vi "一体站流程自动启动.vi"(11 "参数":T1={"是否启用仪器"=FALSE, "CODMn"={"启动测量模式"={"测量模式"=enum."水样测量"}, "确定按钮"=TRUE}, "CODCr"={"启动测量模式"={"测量模式"=enum."水样测量"}}, "采水模式"=enum."使用采水泵"}) -> ()   [LabVIEW 2016, in "PLC.lvlib"]
uses:
  PLC.lvlib
  API/CodCr/CodCr.lvlib
panel:
  out "枚举":enum16{"初始化", "采配水启动", "等待", "配水", "排水", "结束"}(ring)
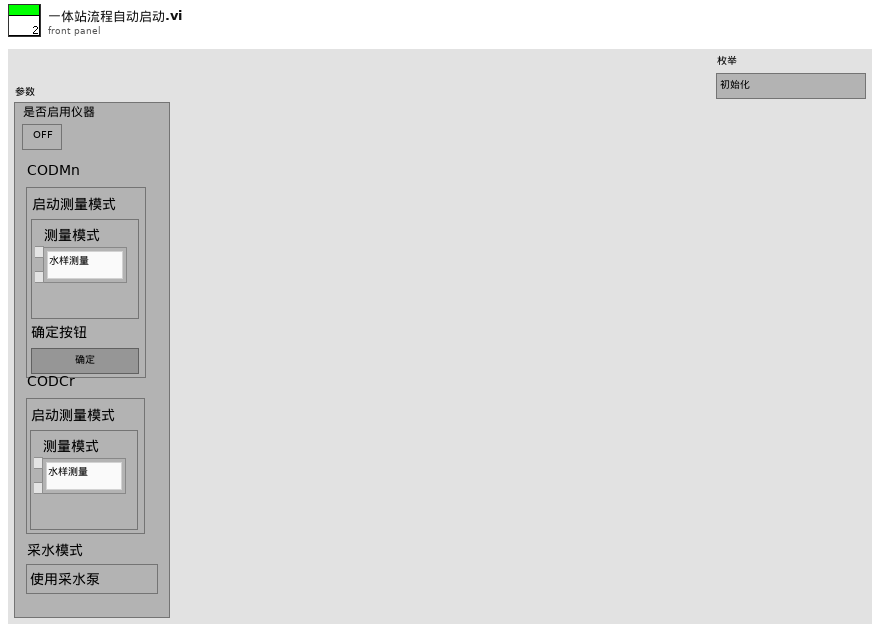
[diagram p1: front panel]
types:
  T1 = cluster{"是否启用仪器":bool, "CODMn":cluster{"启动测量模式":cluster{"测量模式":enum16{"水样测量", "标样核查", "零点核查", "加标回收", "平行样", "校零", "校标"}}, "确定按钮":bool}, "CODCr":cluster{"启动测量模式":cluster{"测量模式":enum16{"水样测量", "标样核查", "零点核查", "加标回收", "平行样", "校零", "校标"}}}, "采水模式":enum16{"使用采水泵", "不使用采水泵"}}
  T2 = cluster{"命令":string, cluster{"starting address":u16, "holding register value":u16}}
  T3 = enum16{"待机", "启动氨氮", "氨氮测量中", "启动总磷", "总磷测量中", "结束"}
  T4 = enum16{"空闲", "水样测试", "标样核查", "零点核查", "跨度核查", "空白测试", "平行样测试", "加标回收", "空白校准", "标样校准", "初始化（清洗）"}
  T5 = cluster{"站号":u16, "量程切换":enum32{"H", "L", "AUTO"}, "控制命令":enum16{"启动测量", "标样核查", "零点核查", "跨度核查", "空白测试", "平行样测试", "加标回收", "空白校准", "标样校准", "初始化（清洗）", "停止测试", "仪器重启", "校时", "模式设置", "测量间隔设置", "盲样测试"}, "模式设置":enum16{"待机", "连续模式", "周期模式", "定点模式", "受控模式", "手动模式"}, "测量间隔":u16}
  T6 = cluster{"时间标识":timestamp, "设备":string, "日志信息":string}
  T7 = cluster{"测试时间":dbl, "运行模式":enum16{"维护模式", "常规模式", "应急模式", "质控模式"}}
  T8 = cluster{"R0":i16, "R1":i16, "R2":i16, "R3":i16, "R4":i16, "R5":i16, "R6":i16, "R7":i16, "R8":i16, "R9":i16, "R10":i16, "R11":i16, "R12":i16, "R13":i16, "R14":i16, "R15":i16, "R16":i16, "R17":i16, "R18":i16, "R19":i16, "R20":i16, "R21":i16}
  T9 = cluster{"测量模式":enum16{"水样测量", "标样核查", "零点核查", "加标回收", "平行样", "校零", "校标"}}
  T10 = enum32{"Bad", "Idle", "Run top level", "Running"}
  T11 = cluster{"系统时间":timestamp, "工作状态":enum16{"空闲", "水样测试", "标样核查", "零点核查", "跨度核查", "空白测试", "平行样测试", "加标回收", "空白校准", "标样校准", "初始化（清洗）"}, "测量模式":enum16{"待机", "连续模式", "周期模式", "定点模式", "受控模式", "手动模式"}, "告警代码":enum16{"无告警", "缺试剂告警", "缺水样告警", "缺蒸馏水告警", "缺标液告警", "仪表漏液告警", "标定异常告警", "超量程告警", "加热异常", "低试剂预警", "超上限告警", "超下限告警", "仪表内部其他异常", "滴定异常告警", "电极异常告警", "量程切换告警", "参数设置告警", "PH电极电位异常", "电导率电极异常", "浊度光度异常", "溶解氧电极异常", "溶解氧光强异常", "温度异常告警", "PH异常告警", "溶解氧异常告警", "电导率异常告警", "浊度异常告警", "叶绿素异常告警", "藻密度异常告警", "蓝绿藻异常告警", "ORP异常告警", "氨氮异常告警", "清洁刷异常告警", "SD卡异常告警", "蓝牙异常告警", "Wifi异常告警", "流程异常告警"}, "故障代码":enum16{"无故障", "电机故障", "温度故障", "通讯故障", "滴定故障"}, "日志代码":u16, "软件版本":u16, "F0":sgl, "F1":sgl, "F2":sgl, "F3":sgl, "T":sgl, "H":sgl, "id":u16, "flowid":u16, "量程":u16}
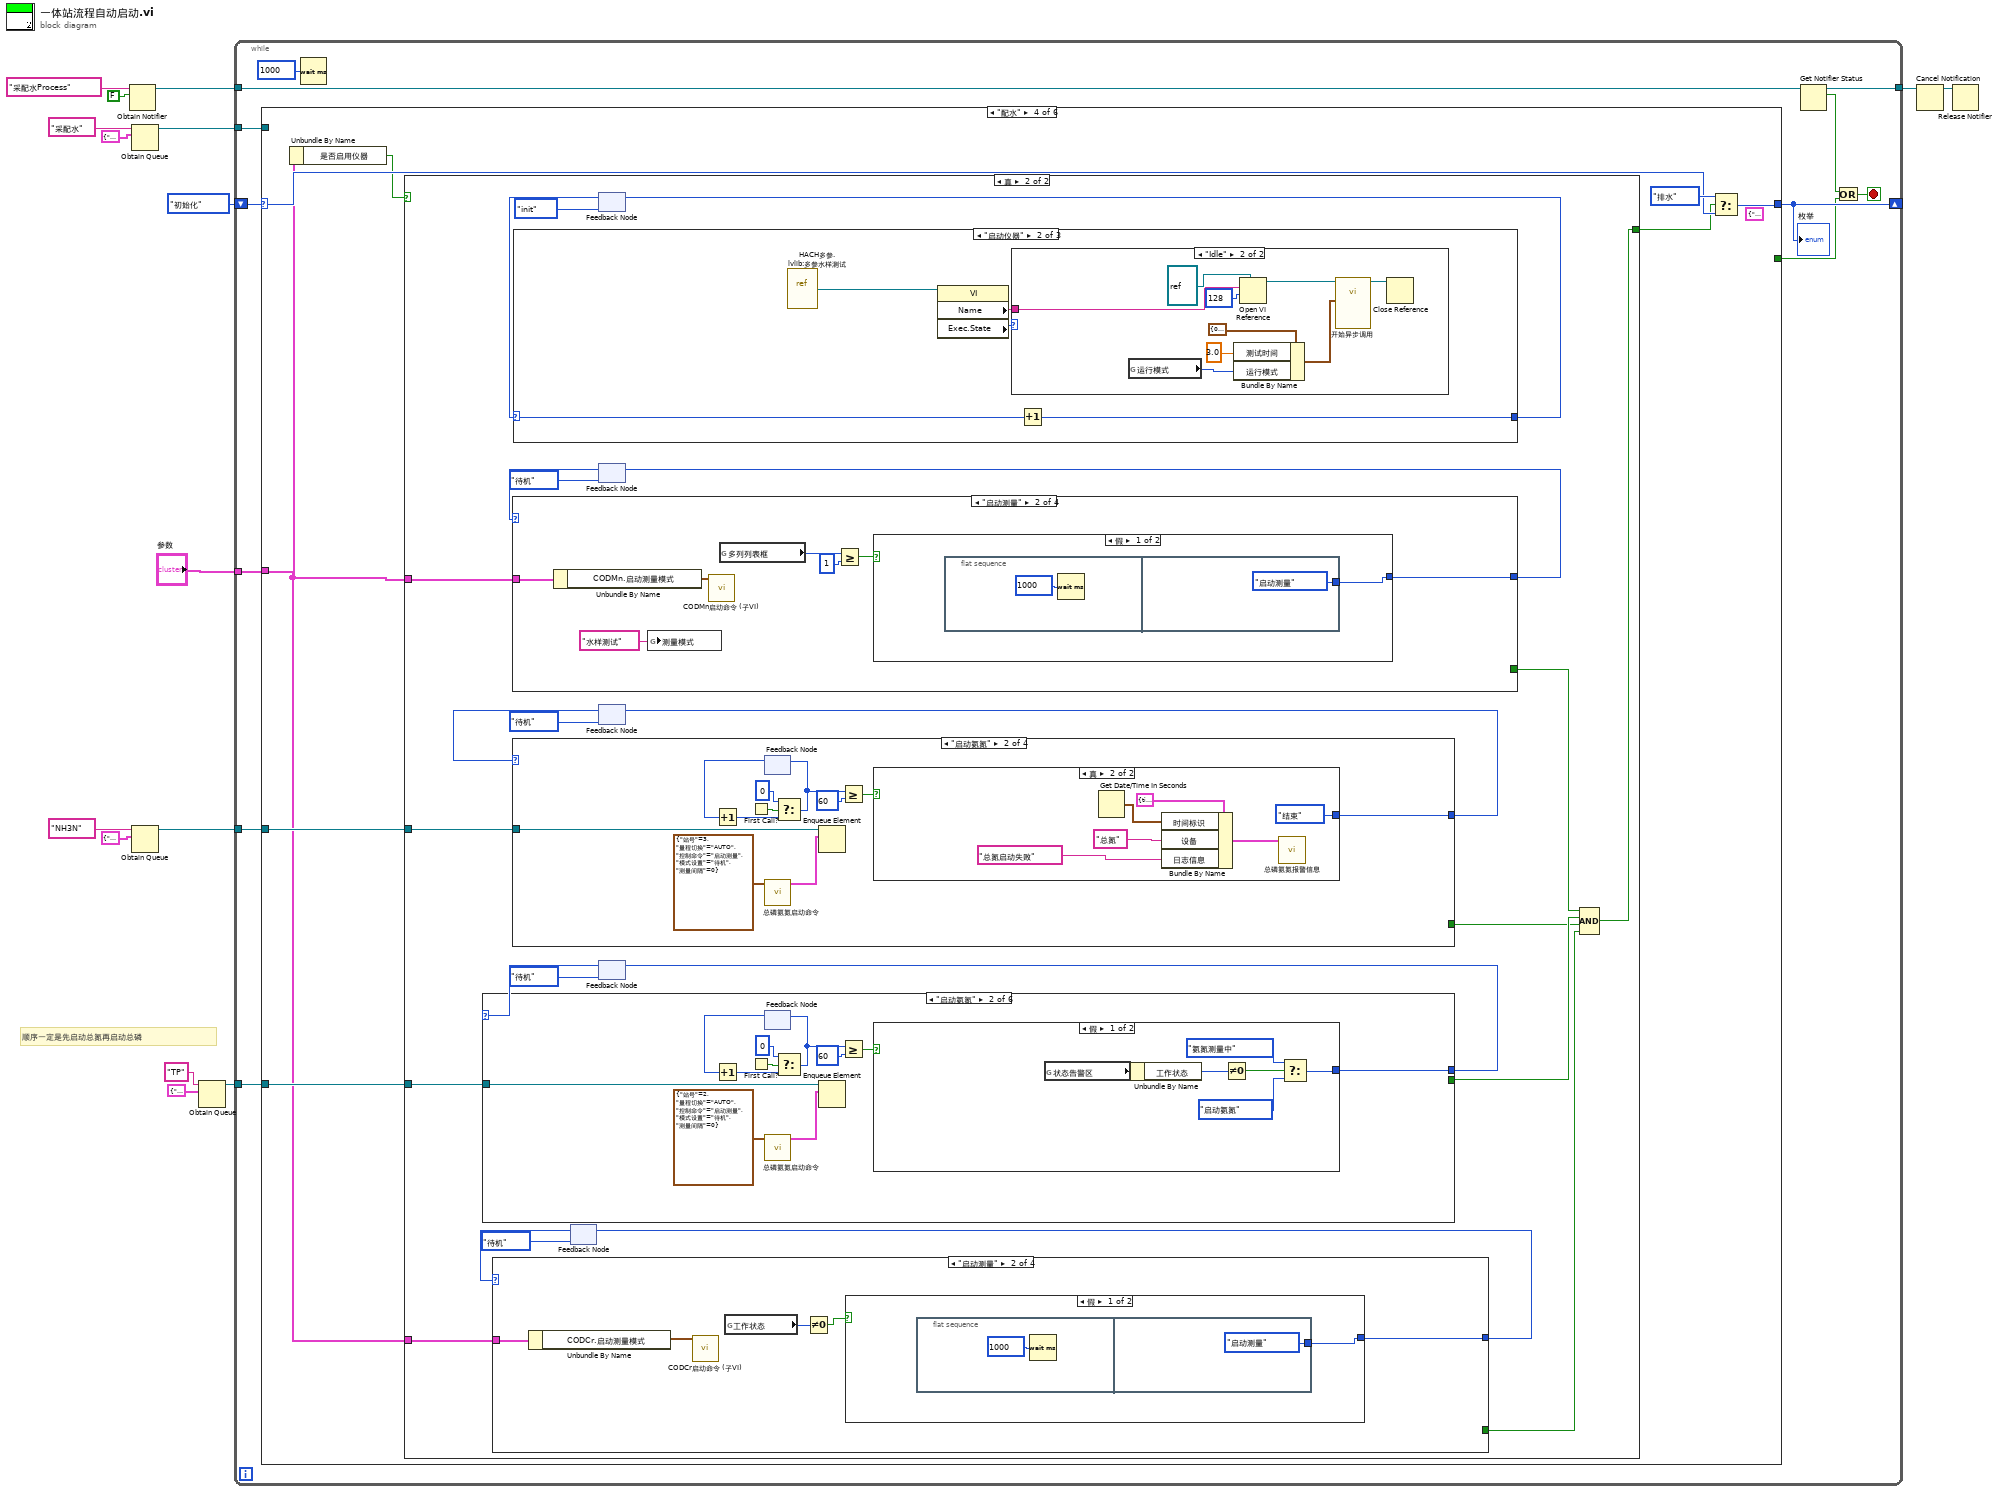
[diagram p0: block diagram]
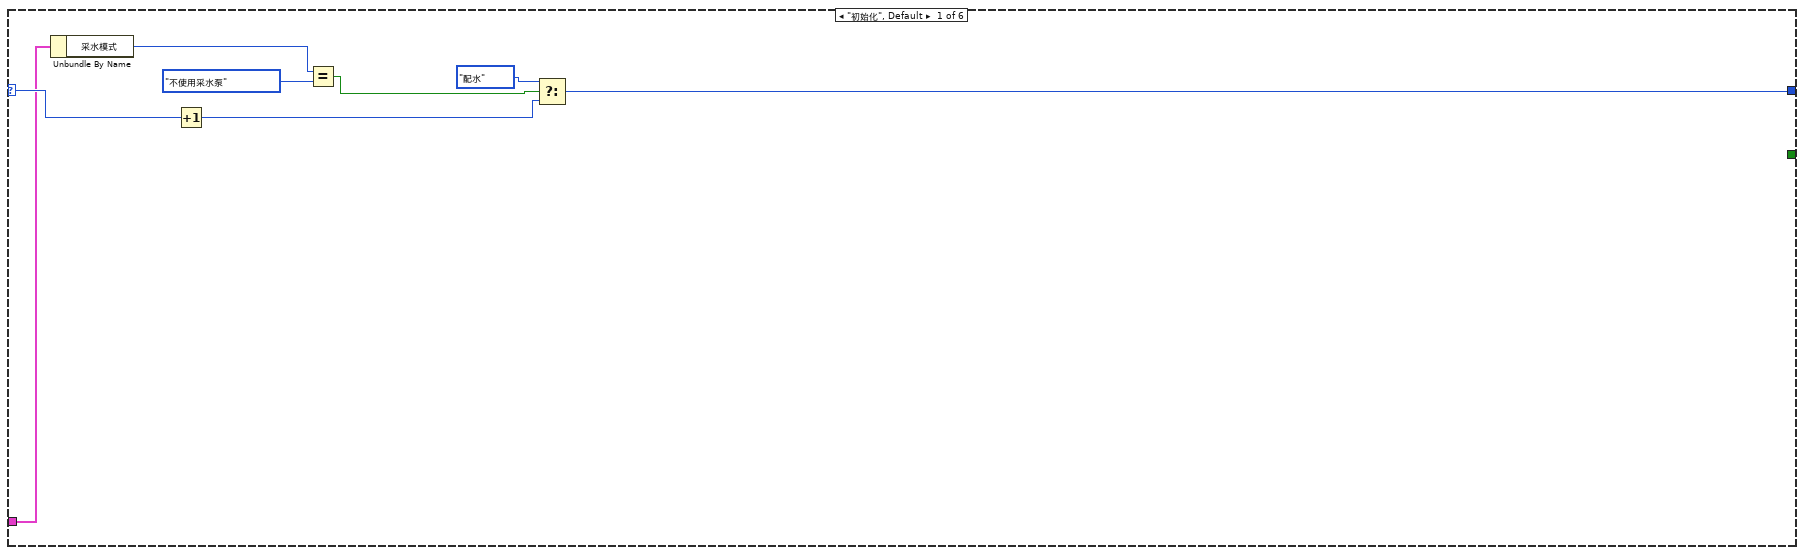
[diagram p2: hidden frame]
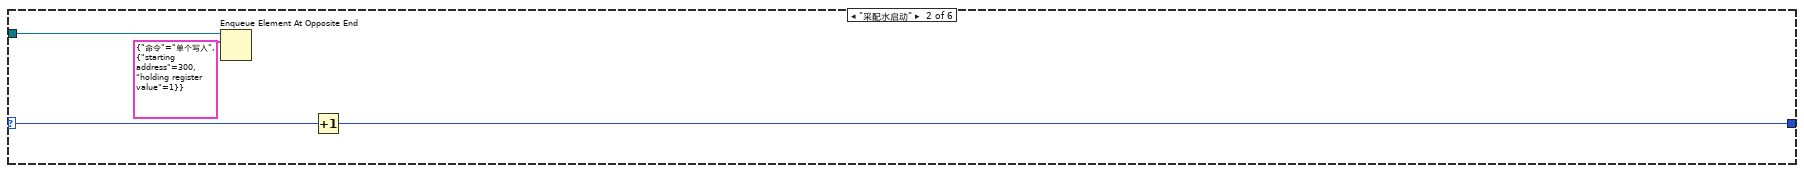
[diagram p3: hidden frame]
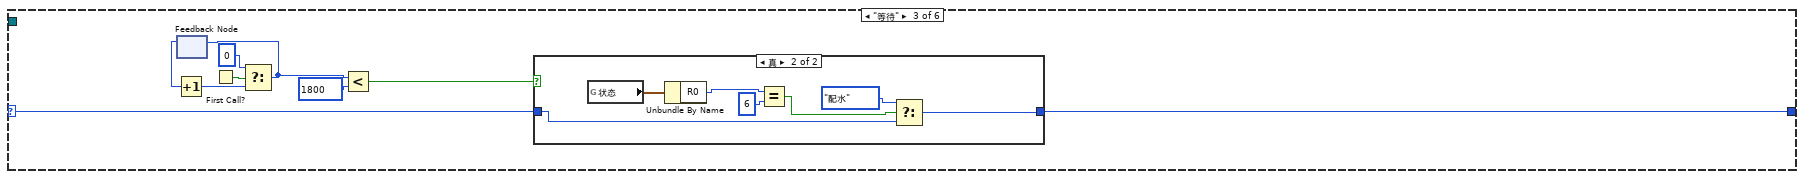
[diagram p4: hidden frame]
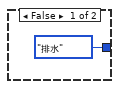
[diagram p5: hidden frame]
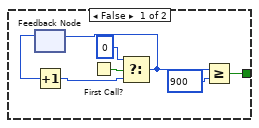
[diagram p6: hidden frame]
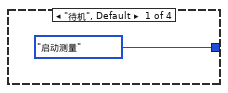
[diagram p7: hidden frame]
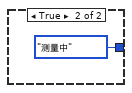
[diagram p8: hidden frame]
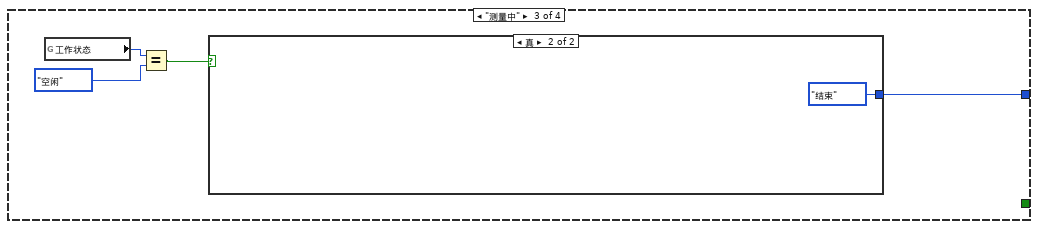
[diagram p9: hidden frame]
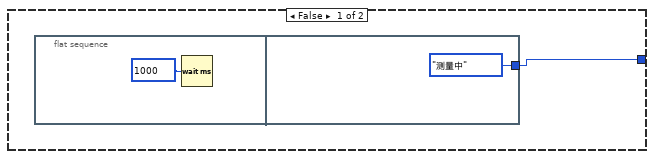
[diagram p10: hidden frame]
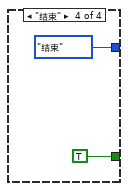
[diagram p11: hidden frame]
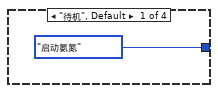
[diagram p12: hidden frame]
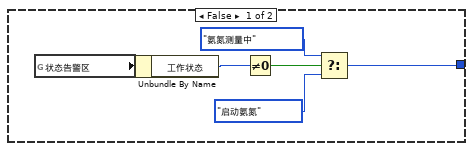
[diagram p13: hidden frame]
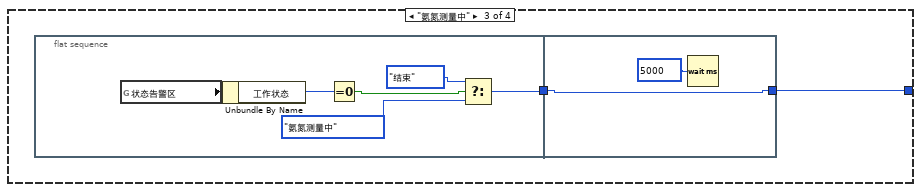
[diagram p14: hidden frame]
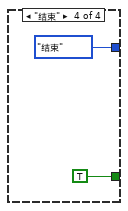
[diagram p15: hidden frame]
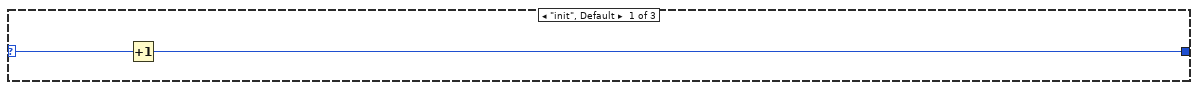
[diagram p16: hidden frame]
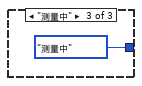
[diagram p18: hidden frame]
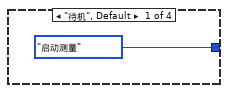
[diagram p19: hidden frame]
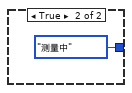
[diagram p20: hidden frame]
diagram:
  # "顺序一定是先启动总氮再启动总磷"
  n1 = Obtain Notifier(name (unnamed)="采配水Process" ("名称（未命名）"), notification data type=FALSE) -> (notifier out=w6:refnum<notifier>)  [unwired: 2 in, 2 out]
  n2 = Obtain Queue(name (unnamed)="采配水" ("名称（未命名）"), element data type=cluster{"命令":string, "数据":variant} {"命令"="", "数据"=variant}) -> (queue out=w14:refnum<queue>)  [unwired: 3 in, 2 out]
  n3 = Obtain Queue(name (unnamed)="NH3N" ("名称（未命名）"), element data type=cluster{"命令":string, "data":variant} {"命令"="", "data"=variant}) -> (queue out=w1:refnum<queue>)  [unwired: 3 in, 2 out]
  n4 = Obtain Queue(name (unnamed)="TP" ("名称（未命名）"), element data type=cluster{"命令":string, "data":variant} {"命令"="", "data"=variant}) -> (queue out=w10:refnum<queue>)  [unwired: 3 in, 2 out]
  n5 = while {
    tunnel: w14 -> [w28]
    shift-right: [w26] -> _
    shift-left: enum16{"初始化", "采配水启动", "等待", "配水", "排水", "结束"}."初始化" ("枚举") -> [w27]
    tunnel: w10 -> [w24]
    tunnel: "参数" -> [w23]
    tunnel: w6 -> [w22]
    tunnel: [w21] -> w5
    tunnel: w1 -> [w17]
    stop <- w20 stop-if-true
    n6 = case shown="\"配水\"" w27 {
      selector: w27 -> [w36 w38 w47 w64 w262 w267]
      tunnel: w28 -> [_ w39 _ _ w263 _]
      tunnel: [w29 w37 w46 w63 w261 w266] -> w26
      tunnel: [_ _ _ _ _ TRUE] -> w19
      tunnel: w24 -> [_ _ _ w62 _ _]
      tunnel: w23 -> [w35 _ _ w58 _ _]
      tunnel: w17 -> [_ _ _ w59 _ _]
      frame "初始化", Default {
        n7 = Unbundle By Name(w35) -> ("采水模式"=w34:enum16{"使用采水泵", "不使用采水泵"})
        n8 = Increment(x=w36) -> (x+1=w30:enum16{"初始化", "采配水启动", "等待", "配水", "排水", "结束"})
        n9 = Equal?(x=w34, y=enum16{"使用采水泵", "不使用采水泵"}."不使用采水泵") -> (x = y?=w32:bool)
        n10 = Select(t=enum16{"初始化", "采配水启动", "等待", "配水", "排水", "结束"}."配水" ("枚举"), s=w32, f=w30) -> (s? t:f=w29:enum16{"初始化", "采配水启动", "等待", "配水", "排水", "结束"})
      }
      frame "采配水启动" {
        n11 = Enqueue Element At Opposite End(queue=w39, element=T2 {"命令"="单个写入", {"starting address"=300, "holding register value"=1}} ("元素")) -> ()  [unwired: 2 in, 3 out]
        n12 = Increment(x=w38) -> (x+1=w37:enum16{"初始化", "采配水启动", "等待", "配水", "排水", "结束"})
      }
      frame "等待" {
        n13 = feedback #1() -> (w43:i32)  [unwired: 1 in]
        n14 = Increment(x=w43) -> (x+1=w42:i32)
        n15 = First Call?() -> (First Call?: T/F=w44:bool)
        n16 = Select(t=0, s=w44, f=w42) -> (s? t:f=w41:i32)
        n17 = feedback-in #1(w41) -> ()
        n18 = Less?(x=w41, y=1800) -> (x < y?=w48:bool)
        n19 = case shown="真" w48 {
          tunnel: w47 -> [_ w52]
          tunnel: [enum16{"初始化", "采配水启动", "等待", "配水", "排水", "结束"}."排水" ("枚举") w51] -> w46
          frame False {
          }
          frame True {
            n20 = global read "采配水全局变量.vi" "状态"() -> (w57:T8)
            n21 = Unbundle By Name(w57) -> ("R0"=w56:i16)
            n22 = Equal?(x=w56, y=i16 6) -> (x = y?=w54:bool)
            n23 = Select(t=enum16{"初始化", "采配水启动", "等待", "配水", "排水", "结束"}."配水" ("枚举"), s=w54, f=w52) -> (s? t:f=w51:enum16{"初始化", "采配水启动", "等待", "配水", "排水", "结束"})
          }
        }
      }
      frame "配水" {
        (unwired) cluster{"命令":string, "data":variant} {"命令"="启动", "data"=variant(cluster{"站号":u16, "控制命令输出":u16[]} {"站号"=1, "控制命令输出"=[256, 0]})} ("元素")
        n24 = Unbundle By Name(w58) -> ("是否启用仪器"=w61:bool)
        n25 = case shown="真" w61 {
          tunnel: w62 -> [_ w93]
          tunnel: [w66 w78] -> w60
          tunnel: w58 -> [_ w89]
          tunnel: w59 -> [_ w82]
          tunnel: w58 -> [_ w74]
          frame False {
            n26 = feedback #2() -> (w70:i32)  [unwired: 1 in]
            n27 = Increment(x=w70) -> (x+1=w69:i32)
            n28 = First Call?() -> (First Call?: T/F=w71:bool)
            n29 = Select(t=0, s=w71, f=w69) -> (s? t:f=w67:i32)
            n30 = feedback-in #2(w67) -> ()
            n31 = Greater Or Equal?(x=w67, y=900) -> (x >= y?=w66:bool)
          }
          frame True {
            n32 = feedback #3(enum16{"待机", "启动测量", "测量中", "结束"}."待机") -> (w76:enum16{"待机", "启动测量", "测量中", "结束"})
            n33 = case shown="\"启动测量\"" w76 {
              tunnel: [enum16{"待机", "启动测量", "测量中", "结束"}."启动测量" w101 w110 enum16{"待机", "启动测量", "测量中", "结束"}."结束"] -> w77
              tunnel: w74 -> [_ w102 _ _]
              tunnel: [_ _ _ TRUE] -> w73
              frame "待机", Default {
              }
              frame "启动测量" {
                n34 = Unbundle By Name(w102) -> ("CODCr.启动测量模式"=w100:T9)
                n35 = call "CODCr启动命令 (子VI).vi"("启动测量模式"=w100) -> ()  [unwired: 11 in]
                n36 = global read "CODCr工作状态.vi" "工作状态"() -> (w99:T4)
                n37 = Not Equal To 0?(x=w99) -> (x != 0?=w98:bool)
                n38 = case shown="假" w98 {
                  tunnel: [w103 enum16{"待机", "启动测量", "测量中", "结束"}."测量中"] -> w101
                  frame False {
                    n39 = flat-sequence {
                      tunnel: [enum16{"待机", "启动测量", "测量中", "结束"}."启动测量"] -> w103
                      frame #0 {
                        n40 = Wait (ms)(milliseconds to wait=u32 1000 ("等待时间（毫秒）")) -> ()  [unwired: 1 out]
                      }
                      frame #1 {
                      }
                    }
                  }
                  frame True {
                  }
                }
              }
              frame "测量中" {
                n41 = global read "CODCr工作状态.vi" "工作状态"() -> (w109:T4)
                n42 = Equal?(x=w109, y=T4."空闲" ("工作状态")) -> (x = y?=w107:bool)
                n43 = case shown="真" w107 {
                  tunnel: [w111 enum16{"待机", "启动测量", "测量中", "结束"}."结束"] -> w110
                  frame False {
                    n44 = flat-sequence {
                      tunnel: [enum16{"待机", "启动测量", "测量中", "结束"}."测量中"] -> w111
                      frame #0 {
                        n45 = Wait (ms)(milliseconds to wait=u32 1000 ("等待时间（毫秒）")) -> ()  [unwired: 1 out]
                      }
                      frame #1 {
                      }
                    }
                  }
                  frame True {
                  }
                }
              }
              frame "结束" {
              }
            }
            n46 = feedback-in #3(w77) -> ()
            n47 = feedback #4(enum16{"init", "启动仪器", "测量中"}."init") -> (w87:enum16{"init", "启动仪器", "测量中"})
            n48 = case shown="\"启动仪器\"" w87 {
              selector: w87 -> [w154 w159 _]
              tunnel: [w153 w158 enum16{"init", "启动仪器", "测量中"}."测量中"] -> w88
              frame "init", Default {
                n49 = Increment(x=w154) -> (x+1=w153:enum16{"init", "启动仪器", "测量中"})
              }
              frame "启动仪器" {
                n50 = vi-ref "HACH多参.lvlib:多参水样测试.vi"() -> (w156:refnum<vi>)
                n51 = property class="VI"(reference=w156) -> ("Name"=w155:string, "Exec.State"=w157:T10)  [unwired: 1 in, 2 out]
                n52 = case shown="\"Idle\"" w157 {
                  tunnel: w155 -> [_ w166]
                  frame "Bad", Default {
                  }
                  frame "Idle" {
                    n53 = global read "系统变量.vi" "运行模式"() -> (w160:enum16{"维护模式", "常规模式", "应急模式", "质控模式"})
                    n54 = Bundle By Name(cluster=T7 {"测试时间"=0.0, "运行模式"=enum."维护模式"} ("API"), "测试时间"=3.0 ("测量时间"), "运行模式"=w160) -> (w162:T7)
                    n55 = Open VI Reference(type specifier VI Refnum (for type only)=refnum<vi> refnum ("类型说明符VI引用句柄（仅用于类型）"), vi path=w166, options=128 ("选项")) -> (vi reference=w165:refnum<vi>)  [unwired: 3 in, 1 out]
                    n56 = call-by-ref "开始异步调用"(reference=w165, "API"=w162) -> (reference out=w164:refnum<vi>)  [unwired: 12 in, 1 out]
                    n57 = Close Reference(reference=w164) -> ()  [unwired: 1 in, 1 out]
                  }
                }
                n58 = Increment(x=w159) -> (x+1=w158:enum16{"init", "启动仪器", "测量中"})
              }
              frame "测量中" {
              }
            }
            n59 = feedback-in #4(w88) -> ()
            n60 = feedback #5(enum16{"待机", "启动测量", "测量中", "结束"}."待机") -> (w91:enum16{"待机", "启动测量", "测量中", "结束"})
            n61 = case shown="\"启动测量\"" w91 {
              tunnel: [enum16{"待机", "启动测量", "测量中", "结束"}."启动测量" w174 w183 enum16{"待机", "启动测量", "测量中", "结束"}."结束"] -> w90
              tunnel: w89 -> [_ w177 _ _]
              tunnel: [_ _ _ TRUE] -> w81
              frame "待机", Default {
              }
              frame "启动测量" {
                n62 = Unbundle By Name(w177) -> ("CODMn.启动测量模式"=w172:T9)
                n63 = global write "COD测量模式全局.vi" "测量模式"("水样测试" ("测量模式")) -> ()
                n64 = call "CODMn启动命令 (子VI).vi"("启动测量模式"=w172) -> ()  [unwired: 11 in]
                n65 = global read "运行时序全局变量.vi" "多列列表框"() -> (w173:i32)
                n66 = Greater Or Equal?(x=w173, y=1) -> (x >= y?=w175:bool)
                n67 = case shown="假" w175 {
                  tunnel: [w178 enum16{"待机", "启动测量", "测量中", "结束"}."测量中"] -> w174
                  frame False {
                    n68 = flat-sequence {
                      tunnel: [enum16{"待机", "启动测量", "测量中", "结束"}."启动测量"] -> w178
                      frame #0 {
                        n69 = Wait (ms)(milliseconds to wait=u32 1000 ("等待时间（毫秒）")) -> ()  [unwired: 1 out]
                      }
                      frame #1 {
                      }
                    }
                  }
                  frame True {
                  }
                }
              }
              frame "测量中" {
                n70 = global read "运行时序全局变量.vi" "多列列表框"() -> (w182:i32)
                n71 = Greater Or Equal?(x=w182, y=5) -> (x >= y?=w184:bool)
                n72 = case shown="真" w184 {
                  tunnel: [w186 enum16{"待机", "启动测量", "测量中", "结束"}."结束"] -> w183
                  frame False {
                    n73 = flat-sequence {
                      tunnel: [enum16{"待机", "启动测量", "测量中", "结束"}."测量中"] -> w186
                      frame #0 {
                        n74 = Wait (ms)(milliseconds to wait=u32 1000 ("等待时间（毫秒）")) -> ()  [unwired: 1 out]
                      }
                      frame #1 {
                      }
                    }
                  }
                  frame True {
                  }
                }
              }
              frame "结束" {
              }
            }
            n75 = feedback-in #5(w90) -> ()
            n76 = feedback #6(T3."待机") -> (w84:T3)
            n77 = case shown="\"启动氨氮\"" w84 {
              tunnel: [T3."启动氨氮" w127 w142 T3."结束"] -> w85
              tunnel: w82 -> [_ w128 _ _]
              tunnel: [_ _ _ TRUE] -> w79
              frame "待机", Default {
              }
              frame "启动氨氮" {
                n78 = First Call?() -> (First Call?: T/F=w125:bool)
                n79 = feedback #7() -> (w124:i32)  [unwired: 1 in]
                n80 = Increment(x=w124) -> (x+1=w123:i32)
                n81 = call "总磷氨氮启动命令.vi"("参数"=T5 {"站号"=3, "量程切换"=enum."AUTO", "控制命令"=enum."启动测量", "模式设置"=enum."待机", "测量间隔"=0}) -> ("启动命令"=w119:cluster{"命令":string, "data":variant})  [unwired: 10 in]
                n82 = Select(t=0, s=w125, f=w123) -> (s? t:f=w122:i32)
                n83 = feedback-in #7(w122) -> ()
                n84 = Enqueue Element(queue=w128, element=w119) -> ()  [unwired: 2 in, 3 out]
                n85 = Greater Or Equal?(x=w122, y=60) -> (x >= y?=w120:bool)
                n86 = case shown="真" w120 {
                  tunnel: [w131 T3."结束"] -> w127
                  frame False {
                    n87 = global read "VAR总磷氨氮全局变量.vi" "状态告警区"() -> (w134:T11)
                    n88 = Unbundle By Name(w134) -> ("工作状态"=w133:T4)
                    n89 = Not Equal To 0?(x=w133) -> (x != 0?=w132:bool)
                    n90 = Select(t=T3."氨氮测量中", s=w132, f=T3."启动氨氮") -> (s? t:f=w131:T3)
                  }
                  frame True {
                    n91 = Get Date/Time In Seconds() -> (seconds since 1Jan1904=w139:timestamp)
                    n92 = Bundle By Name(cluster=T6 {"时间标识"=timestamp(0 s since 1904-01-01), "设备"="", "日志信息"=""} ("data in"), "时间标识"=w139, "设备"="总氮", "日志信息"="总氮启动失败") -> (w135:T6)
                    n93 = call "总磷氨氮报警信息.vi"("data in"=w135) -> ()  [unwired: 11 in]
                  }
                }
              }
              frame "氨氮测量中" {
                n94 = flat-sequence {
                  tunnel: [w146] -> w141
                  tunnel: [w150] -> w142
                  tunnel: w141 -> [w150]
                  frame #0 {
                    n95 = global read "VAR总磷氨氮全局变量.vi" "状态告警区"() -> (w147:T11)
                    n96 = Unbundle By Name(w147) -> ("工作状态"=w148:T4)
                    n97 = Equal To 0?(x=w148) -> (x = 0?=w145:bool)
                    n98 = Select(t=T3."结束", s=w145, f=T3."氨氮测量中") -> (s? t:f=w146:T3)
                  }
                  frame #1 {
                    n99 = Wait (ms)(milliseconds to wait=u32 5000 ("等待时间（毫秒）")) -> ()  [unwired: 1 out]
                  }
                }
              }
              frame "结束" {
              }
            }
            n100 = feedback-in #6(w85) -> ()
            n101 = feedback #8(T3."待机") -> (w95:T3)
            n102 = case shown="\"启动氨氮\"" w95 {
              tunnel: [T3."启动氨氮" w202 w216 w235 w249 T3."结束"] -> w94
              tunnel: w93 -> [_ w203 _ w236 _ _]
              tunnel: [_ _ _ _ _ TRUE] -> w80
              frame "待机", Default {
              }
              frame "启动氨氮" {
                n103 = First Call?() -> (First Call?: T/F=w200:bool)
                n104 = feedback #9() -> (w199:i32)  [unwired: 1 in]
                n105 = Increment(x=w199) -> (x+1=w198:i32)
                n106 = call "总磷氨氮启动命令.vi"("参数"=T5 {"站号"=2, "量程切换"=enum."AUTO", "控制命令"=enum."启动测量", "模式设置"=enum."待机", "测量间隔"=0}) -> ("启动命令"=w194:cluster{"命令":string, "data":variant})  [unwired: 10 in]
                n107 = Select(t=0, s=w200, f=w198) -> (s? t:f=w197:i32)
                n108 = feedback-in #9(w197) -> ()
                n109 = Enqueue Element(queue=w203, element=w194) -> ()  [unwired: 2 in, 3 out]
                n110 = Greater Or Equal?(x=w197, y=60) -> (x >= y?=w195:bool)
                n111 = case shown="假" w195 {
                  tunnel: [w206 T3."启动总磷"] -> w202
                  frame False {
                    n112 = global read "VAR总磷氨氮全局变量.vi" "状态告警区"() -> (w209:T11)
                    n113 = Unbundle By Name(w209) -> ("工作状态"=w208:T4)
                    n114 = Not Equal To 0?(x=w208) -> (x != 0?=w207:bool)
                    n115 = Select(t=T3."氨氮测量中", s=w207, f=T3."启动氨氮") -> (s? t:f=w206:T3)
                  }
                  frame True {
                    n116 = Get Date/Time In Seconds() -> (seconds since 1Jan1904=w214:timestamp)
                    n117 = Bundle By Name(cluster=T6 {"时间标识"=timestamp(0 s since 1904-01-01), "设备"="", "日志信息"=""} ("data in"), "时间标识"=w214, "设备"="总氮", "日志信息"="总氮启动失败") -> (w210:T6)
                    n118 = call "总磷氨氮报警信息.vi"("data in"=w210) -> ()  [unwired: 11 in]
                  }
                }
              }
              frame "氨氮测量中" {
                n119 = global read "VAR总磷氨氮全局变量.vi" "状态告警区"() -> (w219:T11)
                n120 = Unbundle By Name(w219) -> ("工作状态"=w217:T4, "id"=w218:u16)
                n121 = case shown="\"空闲\"" w217 {
                  tunnel: w218 -> [_ w223]
                  tunnel: [T3."启动总磷" w222] -> w216
                  frame "空闲" {
                    n122 = Wait (ms)(milliseconds to wait=u32 8000 ("等待时间（毫秒）")) -> ()  [unwired: 1 out]
                  }
                  frame Default {
                    n123 = case shown="131" w223 {
                      tunnel: [T3."氨氮测量中" T3."总磷测量中"] -> w222
                      frame 76, Default {
                      }
                      frame 131 {
                      }
                    }
                  }
                }
              }
              frame "启动总磷" {
                n124 = First Call?() -> (First Call?: T/F=w233:bool)
                n125 = feedback #10() -> (w232:i32)  [unwired: 1 in]
                n126 = Increment(x=w232) -> (x+1=w231:i32)
                n127 = call "总磷氨氮启动命令.vi"("参数"=T5 {"站号"=1, "量程切换"=enum."AUTO", "控制命令"=enum."启动测量", "模式设置"=enum."待机", "测量间隔"=0}) -> ("启动命令"=w227:cluster{"命令":string, "data":variant})  [unwired: 10 in]
                n128 = Select(t=0, s=w233, f=w231) -> (s? t:f=w230:i32)
                n129 = feedback-in #10(w230) -> ()
                n130 = Enqueue Element(queue=w236, element=w227) -> ()  [unwired: 2 in, 3 out]
                n131 = Greater Or Equal?(x=w230, y=60) -> (x >= y?=w228:bool)
                n132 = case shown="真" w228 {
                  tunnel: [w239 T3."结束"] -> w235
                  frame False {
                    n133 = global read "VAR总磷氨氮全局变量.vi" "状态告警区"() -> (w240:T11)
                    n134 = Unbundle By Name(w240) -> ("工作状态"=w241:T4)
                    n135 = Not Equal To 0?(x=w241) -> (x != 0?=w242:bool)
                    n136 = Select(t=T3."总磷测量中", s=w242, f=T3."启动总磷") -> (s? t:f=w239:T3)
                  }
                  frame True {
                    n137 = Get Date/Time In Seconds() -> (seconds since 1Jan1904=w248:timestamp)
                    n138 = Bundle By Name(cluster=T6 {"时间标识"=timestamp(0 s since 1904-01-01), "设备"="", "日志信息"=""} ("data in"), "时间标识"=w248, "设备"="总磷", "日志信息"="总磷启动失败") -> (w243:T6)
                    n139 = call "总磷氨氮报警信息.vi"("data in"=w243) -> ()  [unwired: 11 in]
                  }
                }
              }
              frame "总磷测量中" {
                n140 = global read "VAR总磷氨氮全局变量.vi" "状态告警区"() -> (w252:T11)
                n141 = Unbundle By Name(w252) -> ("工作状态"=w250:T4, "id"=w251:u16)
                n142 = case shown="\"空闲\"" w250 {
                  tunnel: w251 -> [_ w256]
                  tunnel: [T3."结束" w255] -> w249
                  frame "空闲" {
                    n143 = Wait (ms)(milliseconds to wait=u32 8000 ("等待时间（毫秒）")) -> ()  [unwired: 1 out]
                  }
                  frame Default {
                    n144 = case shown="131" w256 {
                      tunnel: [T3."氨氮测量中" T3."总磷测量中"] -> w255
                      frame 76, Default {
                      }
                      frame 131 {
                      }
                    }
                  }
                }
              }
              frame "结束" {
              }
            }
            n145 = feedback-in #8(w94) -> ()
            n146 = Compound Arithmetic op=AND ("复合运算")(w81, w80, w79, w73) -> (w78:bool)
          }
        }
        n147 = Select(t=enum16{"初始化", "采配水启动", "等待", "配水", "排水", "结束"}."排水" ("枚举"), s=w60, f=w64) -> (s? t:f=w63:enum16{"初始化", "采配水启动", "等待", "配水", "排水", "结束"})
      }
      frame "排水" {
        n148 = Enqueue Element At Opposite End(queue=w263, element=T2 {"命令"="单个写入", {"starting address"=303, "holding register value"=1}} ("元素")) -> ()  [unwired: 2 in, 3 out]
        n149 = Increment(x=w262) -> (x+1=w261:enum16{"初始化", "采配水启动", "等待", "配水", "排水", "结束"})
      }
      frame "结束" {
        n150 = Increment(x=w267) -> (x+1=w266:enum16{"初始化", "采配水启动", "等待", "配水", "排水", "结束"})
      }
    }
    "枚举" <- w26
    n151 = Wait (ms)(milliseconds to wait=u32 1000 ("等待时间（毫秒）")) -> ()  [unwired: 1 out]
    n152 = Get Notifier Status(notifier=w22) -> (notifier out=w21:refnum<notifier>, current notification=w18:bool)  [unwired: 1 in, 3 out]
    n153 = Or(x=w18, y=w19) -> (x .or. y?=w20:bool)
  }
  n154 = Cancel Notification(0:w5) -> (8:w4:refnum<notifier>)  [unwired: 1 in, 2 out]
  n155 = Release Notifier(notifier=w4) -> ()  [unwired: 2 in, 3 out]
